vi "Update-sender-activity.vi"(8 "error in (no error)":errorcluster, 10 "Message":refnum<class "Message.lvclass">, 11 "ModComm in":T1) -> (0 "error out":errorcluster, 2 "Message dup":refnum<class "Message.lvclass">, 3 "ModComm out":T1)   [LabVIEW 2013, in "Server.lvlib" / "Server.lvclass"]
uses:
  Server.lvclass
  Object-reference.ctl
  Messages/Sources/Message.lvclass
  Messages/Sources/Message.lvclass/Message.ctl
  Messages/Sources/Read Sender ID.vi
  Messages/Sources/Read Send time.vi
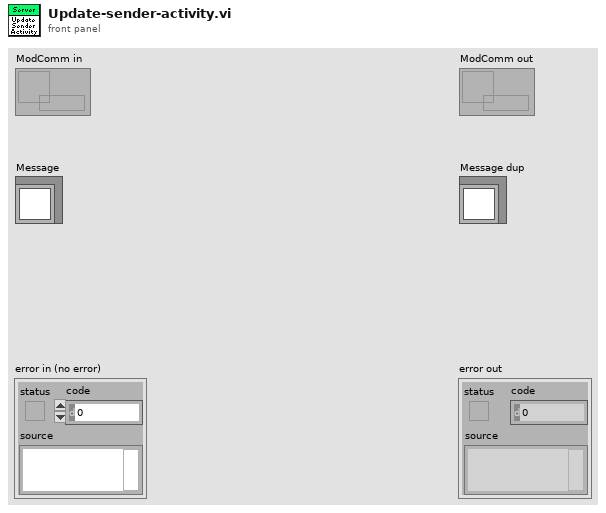
[diagram p1: front panel]
types:
  T1 = typedef "Server.lvlib/Server.lvclass/Object-reference.ctl" = refnum<data-value>
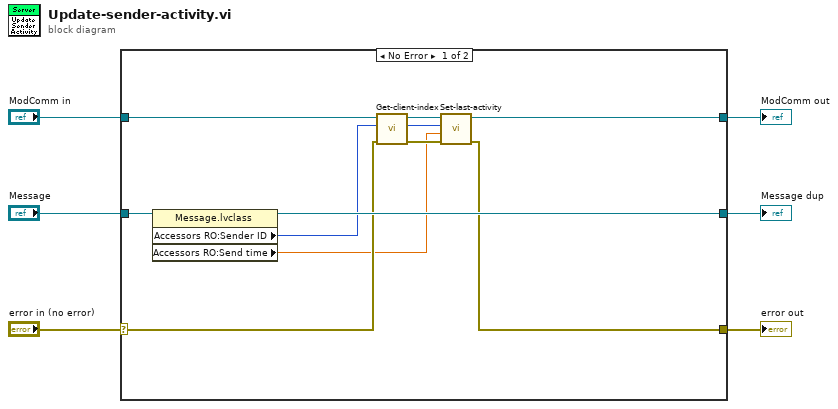
[diagram p0: block diagram]
diagram:
  n1 = case shown="No Error" "error in (no error)" {
    selector: "error in (no error)" -> [w12 w20]
    tunnel: [w11 w20] -> w5
    tunnel: [w14 w19] -> w3
    tunnel: "ModComm in" -> [w15 w19]
    tunnel: "Message" -> [w17 w18]
    tunnel: [w16 w18] -> w1
    frame No Error {
      n2 = property class="Message.lvclass"(reference=w17) -> (reference out=w16:refnum<class "Message.lvclass">, "Accessors RO:Sender ID"=w8:i32, "Accessors RO:Send time"=w7:dbl)  [unwired: 1 in, 1 out]
      n3 = call "Get-client-index.vi"("error in (no error)"=w12, "Client ID"=w8, "ModComm in"=w15) -> ("error out"=w10:errorcluster, "Client index"=w9:i32, "ModComm out"=w13:T1)  [unwired: 6 in]
      n4 = call "Set-last-activity.vi"("error in (no error)"=w10, "Last contact"=w7, "Client index"=w9, "ModComm in"=w13) -> ("error out"=w11:errorcluster, "ModComm out"=w14:T1)  [unwired: 6 in]
    }
    frame Error {
    }
  }
  "error out" <- w5
  "ModComm out" <- w3
  "Message dup" <- w1
